vi "isInitialized.vi"(8 "error in (no error)":errorcluster, 11 "ITaskStopMechanism in":refnum<class "ITaskChannel.lvclass">) -> (0 "error out":errorcluster, 2 "isInitRequired":bool, 3 "ITaskStopMechanism out":refnum<class "ITaskChannel.lvclass">)   [LabVIEW 2023, in "TLC_Daemon.lvlib" / "ITaskChannel.lvclass"]
doc: "Returns False if the StopMechanism requires initialization (so it returns True if the StopMechanism is already initialized).\nThis is useful for handling both of the following cases:\n- Internal Initialization: The StopMechanism is initialized by the TaskController, which handles the entire lifecycle.\n- External Initialization: The StopMechanism is already initialized externally. This is used when you need to share the mechanism with other components (such as message queues).\n\nNote: Use external initialization carefully; the TaskController sends stopRequests, which may impact external code."
uses:
  ITaskChannel.lvclass
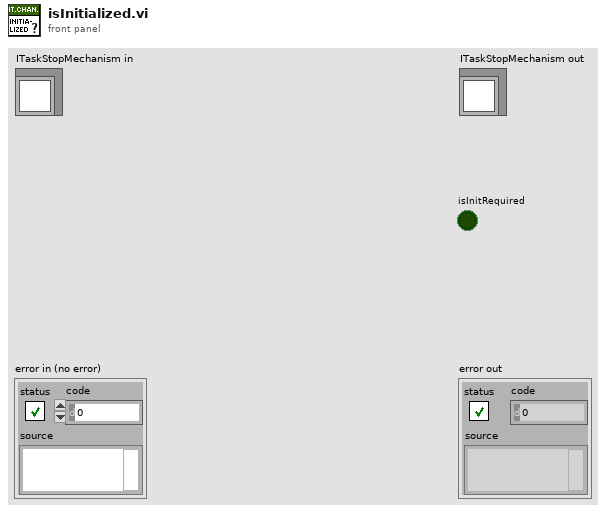
[diagram p1: front panel]
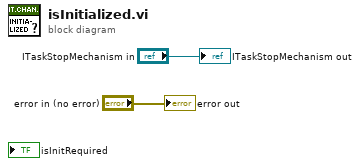
[diagram p0: block diagram]
diagram:
  "error out" <- "error in (no error)"
  "ITaskStopMechanism out" <- "ITaskStopMechanism in"
